vi "Draw Model.vi"(8 "error in (no error)":errorcluster, 10 "Cluster":T1, 11 "SceneObject in":refnum<vi>) -> (0 "error out":errorcluster)   [LabVIEW 2018]
uses:
  <vilib>/picture/3D Picture Control/NI_3D Picture Control.lvlib
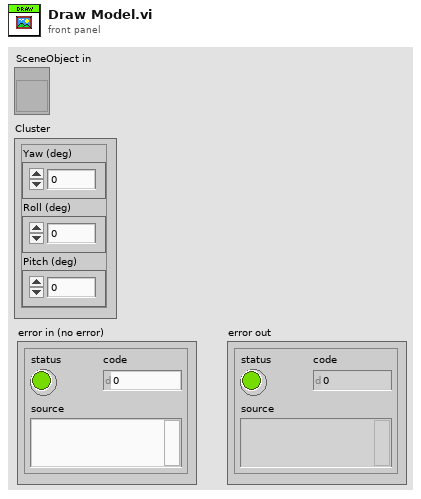
[diagram p1: front panel]
types:
  T1 = cluster{"Yaw (deg)":dbl, "Roll (deg)":dbl, "Pitch (deg)":dbl}
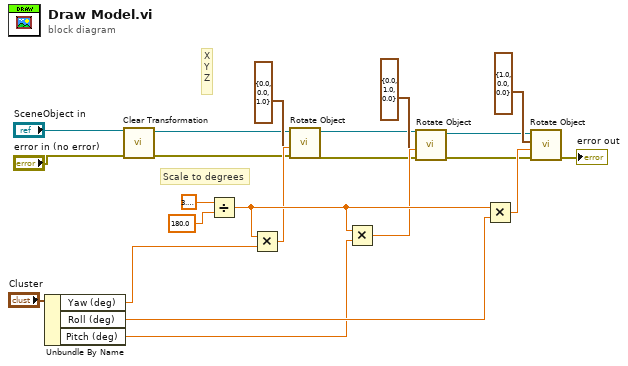
[diagram p0: block diagram]
diagram:
  # "Scale to degrees"
  # "X\nY\nZ"
  n1 = Unbundle By Name("Cluster") -> ("Yaw (deg)"=w1:dbl, "Roll (deg)"=w3:dbl, "Pitch (deg)"=w2:dbl)
  n2 = call <vilib>:"Clear Transformation.vi"("error in (no error)"="error in (no error)", "Object Refnum In"="SceneObject in") -> ("error out"=w6:errorcluster, "Object Refnum Out"=w5:refnum<vi>)  [unwired: 8 in]
  n3 = Divide(x=3.141592653589793, y=180.0) -> (x/y=w19:dbl)
  n4 = Multiply(x=w19, y=w1) -> (x*y=w18:dbl)
  n5 = call <vilib>:"Rotate Object.vi"("error in (no error)"=w6, "Angle"=w18, "Axis"=cluster{"X":sgl, "Y":sgl, "Z":sgl} {"X"=0.0, "Y"=0.0, "Z"=1.0}, "Scene.Object In"=w5) -> ("error out"=w10:errorcluster, "Scene.Object Out"=w7:refnum<vi>)  [unwired: 6 in]
  n6 = Multiply(x=w19, y=w2) -> (x*y=w17:dbl)
  n7 = call <vilib>:"Rotate Object.vi"("error in (no error)"=w10, "Angle"=w17, "Axis"=cluster{"X":sgl, "Y":sgl, "Z":sgl} {"X"=0.0, "Y"=1.0, "Z"=0.0}, "Scene.Object In"=w7) -> ("error out"=w9:errorcluster, "Scene.Object Out"=w8:refnum<vi>)  [unwired: 6 in]
  n8 = Multiply(x=w19, y=w3) -> (x*y=w16:dbl)
  n9 = call <vilib>:"Rotate Object.vi"("error in (no error)"=w9, "Angle"=w16, "Axis"=cluster{"X":sgl, "Y":sgl, "Z":sgl} {"X"=1.0, "Y"=0.0, "Z"=0.0}, "Scene.Object In"=w8) -> ("error out"=→"error out":errorcluster)  [unwired: 6 in, 1 out]
